vi "create.vi"(8 "error in":errorcluster, 10 "max queue size (50)":i32=50, 11 "enqueue mode":T1) -> (0 "error out":errorcluster, 3 "stream publisher out":refnum<class "data bus stream subscriber.lvclass">)   [LabVIEW 2013, in "data bus stream subscriber.lvclass"]
uses:
  data bus stream subscriber.lvclass
  enqueue mode.ctl
  data stream definition.ctl
  data stream message type.ctl
  data bus stream subscriber.lvclass/data bus stream subscriber.ctl
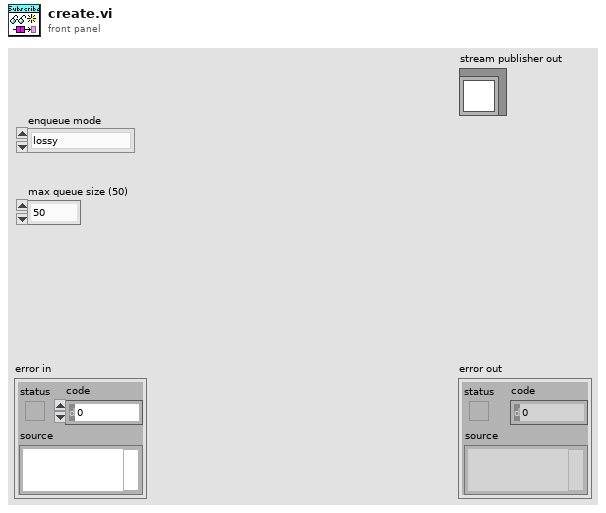
[diagram p1: front panel]
types:
  T1 = typedef "data bus stream subscriber.lvclass/enqueue mode.ctl" = enum16{"lossy", "lossless"}
  T2 = typedef "data stream definition.ctl" = cluster{"contained data":T3, "message name":string, "Waveform":waveform(dbl), "payload":variant}
  T3 = typedef "data stream message type.ctl" = enum16{"waveform", "message"}
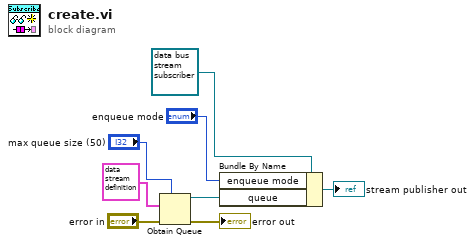
[diagram p0: block diagram]
diagram:
  n1 = Obtain Queue(max queue size (-1, unlimited)="max queue size (50)", element data type=T2 {"contained data"=enum."waveform", "message name"="", "Waveform"={"t0"=timestamp(0 s since 1904-01-01), "dt"=1.0, "Y"=[]}, "payload"=variant} ("stream definition"), error in (no error)="error in") -> (queue out=w2:refnum<queue>, error out=→"error out":errorcluster)  [unwired: 2 in, 1 out]
  n2 = Bundle By Name(cluster=refnum<class "data bus stream subscriber.lvclass"> refnum ("stream publisher in"), "enqueue mode"="enqueue mode", "queue"=w2) -> (→"stream publisher out":refnum<class "data bus stream subscriber.lvclass">)
